vi "FPGA_SICMAutoApproach_v1.vi"() -> ()   [LabVIEW 2021]
uses:
  <vilib>/rvi/eio/common/nirviEmuTemplateMethod_errors.vi
  <vilib>/rvi/Emulation/niFpgaGetClockAttributes.vi
  <vilib>/rvi/Emulation/niFpgaSctlEmulationGetInTimedLoop.vi
  <vilib>/rvi/Emulation/niFpgaEmulationReportErrorSimple.vi
  <vilib>/rvi/Emulation/niFpgaCriticalErrorInLSC.vi
  <vilib>/rvi/Emulation/niFpgaProcessEmulError.vi
  <vilib>/rvi/interface/RandomDataEmulation/niFpgaRandomDataHandleErrors.vi
  <vilib>/rvi/Emulation/niFpgaEmulationIsFPGAContextNoSignature.vi
  <vilib>/rvi/DataTransferAndStorage/Container/Common/niFpgaContainerGetUniqueNameForEmu.vi
  <vilib>/rvi/Memory/Memory_Emulation/niFpgaMemoryEmulationCacheClearOnFirstRun.vi
  <vilib>/rvi/Memory/Memory_Emulation/nirvimemoryEmulationManagerCache_MakeExclusive.vi
  <vilib>/rvi/Memory/Memory_Emulation/niFpgaMemoryEmulationValidateCache.vi
  <vilib>/rvi/Memory/Memory_Emulation/nirvimemoryEmulationManagerCache_InsertValue.vi
  <vilib>/Utility/error.llb/Clear Errors.vi
  <vilib>/rvi/Memory/Memory_Emulation/nirvimemoryEmulationManagerCache_ReleaseExclusive.vi
  <vilib>/rvi/Memory/Memory_Emulation/nirvimemoryEmulationManagerCache_GetValue.vi
  <vilib>/rvi/Memory/Memory_Emulation/nirvimemoryEmulationManagerCache_SetValue.vi
  <vilib>/rvi/occurrence/nirviWaitOnOccurrenceBase.vi
  <vilib>/eio/EIONode/EIONode.xnode
  <vilib>/rvi/FXPMathLib/FxpAdd/XNode/nifxpmath_Add.xnode
  <vilib>/rvi/DataTransferAndStorage/Container/XNode/niFpgaContainer.xnode
  <vilib>/rvi/interface/RandomDataEmulation/nirviRandomDataFpgaReadWriteTemplate.vi
  <vilib>/rvi/DataTransferAndStorage/Register/Emulation/niFpgaRegisterEmulation.vi
  <vilib>/rvi/FXPMathLib/FxpSub/XNode/nifxpmath_Sub.xnode
  <vilib>/rvi/FXPMathLib/sim/FxpSim.dll
panel:
  in  "QuietTime us":u16
  in  "Retract us/step":u32=50
  in  "HoldingElapse us":u32
  in  "SurfaceHold":bool
  out "PeizoFeedbackPos":fxp<+/-,27,5>
  out "PeizoThresholdPos":fxp<+/-,33,17>
  out "PresCurr":fxp<+/-,27,5>
  out "Approached!":bool
  out "ZPeizoPresPos":fxp<+/-,33,17>
  in  "ApproachRate us":u16
  in  "PeizoMax":fxp<+/-,32,16>
  in  "BaselineCurrent":fxp<+/-,32,16>
  in  "stop":bool
  in  "PeizoOffset":fxp<+/-,32,16>
  in  "DeltaMode":bool
  in  "Threshold":fxp<+/-,32,16>
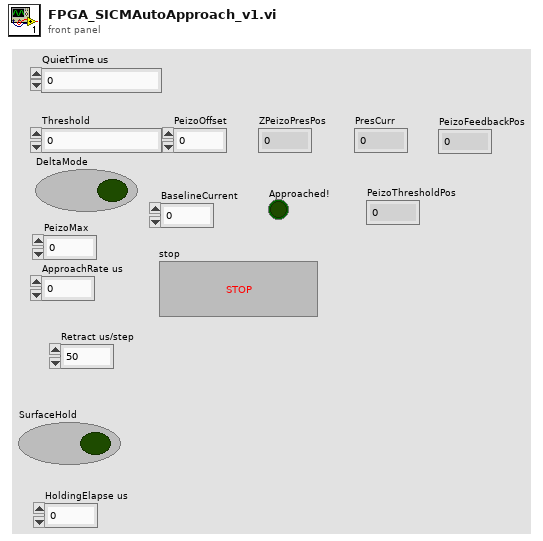
[diagram p1: front panel]
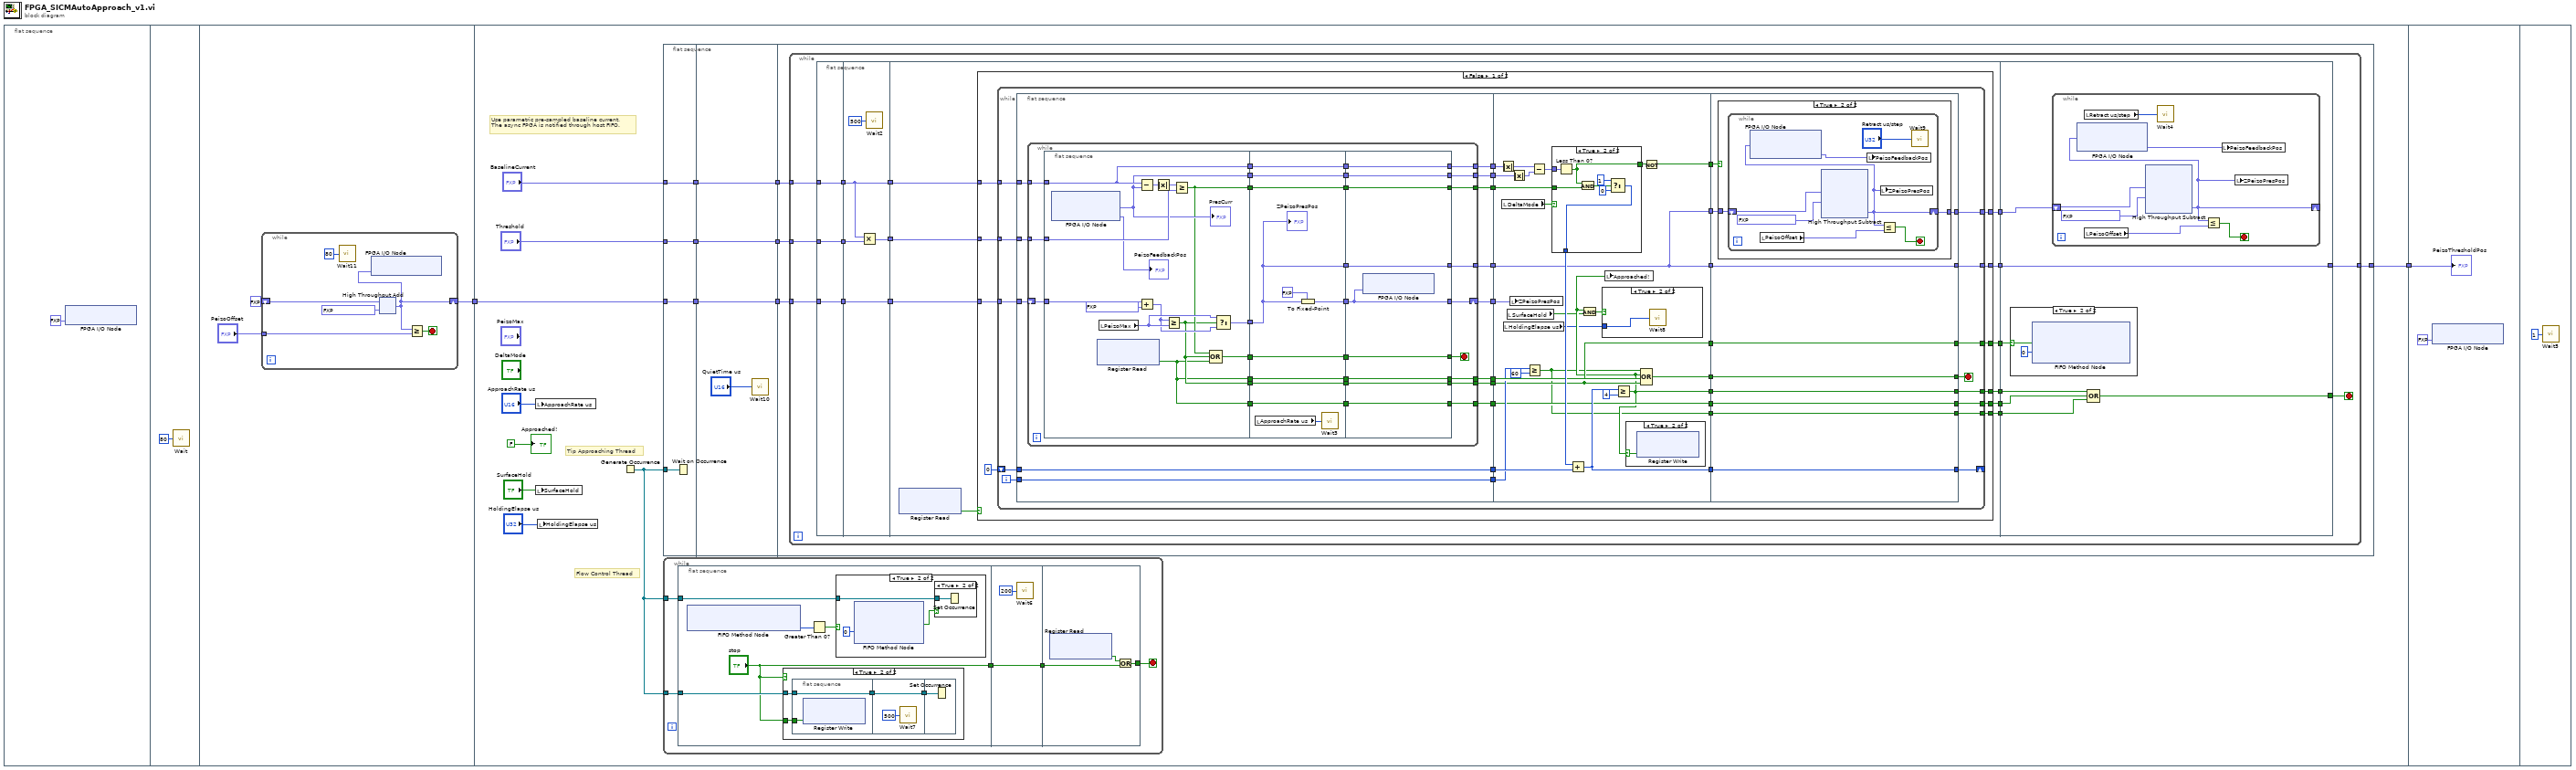
[diagram p0: block diagram]
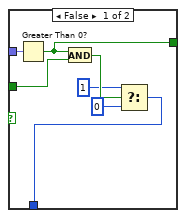
[diagram p4: hidden frame]
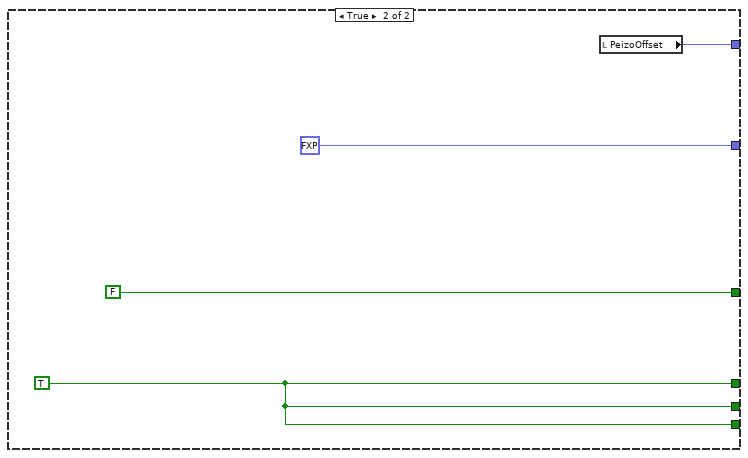
[diagram p6: hidden frame]
diagram:
  n1 = flat-sequence {
    tunnel: [w5] -> w1
    tunnel: [w23] -> w2
    tunnel: w1 -> [w14]
    tunnel: w2 -> [w305]
    frame #0 {
      n2 = xnode "FPGA I/O Node"("Connector0/AO4"=fxp<+/-,20,5> 0.0 ("Connector0/AO2")) -> ()  [unwired: 1 in, 1 out]
    }
    frame #1 {
      n3 = call "Wait"("Count(mSec)"=u8 80) -> ()  [unwired: 1 out]
    }
    frame #2 {
      n4 = while {
        tunnel: "PeizoOffset" -> [w9]
        shift-right: [w10] -> w5
        shift-left: fxp<+/-,48,16> 0.0 -> [w12]
        stop <- w8 stop-if-true
        n5 = call "Wait11"("Count(uSec)"=u32 80) -> ()  [unwired: 1 out]
        n6 = xnode "High Throughput Add"("x"=w12, "y"=fxp<+/-,48,16> 0.00030517578125) -> ("x+y"=w10:fxp<+/-,48,16>)
        n7 = xnode "FPGA I/O Node"("Connector0/AO2"=w10) -> ()  [unwired: 1 in, 1 out]
        n8 = Greater Or Equal?(x=w10, y=w9) -> (x >= y?=w8:bool)
      }
    }
    frame #3 {
      # "Tip Approaching Thread"
      # "Flow Control Thread"
      # "Use parametric pre-sampled baseline current. \nThe async FPGA is notified through host FIFO."
      n9 = local write "ApproachRate us"("ApproachRate us") -> ()
      n10 = local write "SurfaceHold"("SurfaceHold") -> ()
      n11 = local write "HoldingElapse us"("HoldingElapse us") -> ()
      n12 = Generate Occurrence() -> (w28:refnum<k4>)
      n13 = flat-sequence {
        tunnel: "BaselineCurrent" -> [w30]
        tunnel: "Threshold" -> [w31]
        tunnel: w14 -> [w32]
        tunnel: w28 -> [w29]
        tunnel: [w32] -> w17
        tunnel: [w31] -> w16
        tunnel: [w30] -> w15
        tunnel: [w36] -> w20
        tunnel: [w35] -> w19
        tunnel: [w34] -> w18
        tunnel: w17 -> [w36]
        tunnel: w16 -> [w35]
        tunnel: w15 -> [w34]
        tunnel: [w37] -> w23
        tunnel: w20 -> [w40]
        tunnel: w19 -> [w39]
        tunnel: w18 -> [w38]
        frame #0 {
          n14 = Wait on Occurrence(2:w29) -> ()  [unwired: 2 in, 1 out]
        }
        frame #1 {
          n15 = call "Wait10"("Count(uSec)"="QuietTime us") -> ()  [unwired: 1 out]
        }
        frame #2 {
          n16 = while {
            tunnel: w38 -> [w49]
            tunnel: w40 -> [w48]
            tunnel: w39 -> [w47]
            tunnel: [w43] -> w37
            stop <- w51 stop-if-true
            n17 = flat-sequence {
              tunnel: [w60] -> w57
              tunnel: [w59] -> w56
              tunnel: [w58] -> w55
              tunnel: w47 -> [w60]
              tunnel: w48 -> [w58]
              tunnel: w49 -> [w59]
              tunnel: w57 -> [w64]
              tunnel: w56 -> [w63]
              tunnel: [w63] -> w54
              tunnel: w55 -> [w62]
              tunnel: [w62] -> w53
              tunnel: [w61] -> w52
              tunnel: w54 -> [w74]
              tunnel: w53 -> [w73]
              tunnel: w52 -> [w72]
              tunnel: [w71] -> w50
              tunnel: [w70] -> w46
              tunnel: [w69] -> w45
              tunnel: [w68] -> w44
              tunnel: [w67] -> w42
              tunnel: [w66] -> w41
              tunnel: [w266] -> w51
              tunnel: w50 -> [w265]
              tunnel: w46 -> [w267]
              tunnel: w45 -> [w264]
              tunnel: w44 -> [w262]
              tunnel: [w262] -> w43
              tunnel: w42 -> [w263]
              tunnel: w41 -> [w261]
              frame #0 {
              }
              frame #1 {
                n18 = Multiply(x=w63, y=w64) -> (x*y=w61:fxp<+/-,64,32>)
                n19 = call "Wait2"("Count(uSec)"=u16 500) -> ()  [unwired: 1 out]
              }
              frame #2 {
                n20 = xnode ("Register Read")() -> ("Data"=w75:bool)  [unwired: 1 in, 1 out]
                n21 = case shown="False" w75 {
                  tunnel: w74 -> [w85 _]
                  tunnel: w73 -> [w84 _]
                  tunnel: w72 -> [w83 _]
                  tunnel: [w81 w258] -> w71
                  tunnel: [w80 FALSE] -> w70
                  tunnel: [w79 w258] -> w69
                  tunnel: [w78 fxp<+/-,33,17> 0.0 ("PeizoMax")] -> w68
                  tunnel: [w77 w258] -> w67
                  tunnel: [w76 w257] -> w66
                  frame False {
                    n22 = while {
                      tunnel: w85 -> [w116]
                      tunnel: w84 -> [w117]
                      tunnel: w83 -> [w115]
                      shift-right: [w105] -> _
                      shift-left: i16 0 -> [w107]
                      tunnel: [w103] -> w81
                      tunnel: [w96] -> w80
                      tunnel: [w93] -> w79
                      tunnel: [w90] -> w78
                      tunnel: [w88] -> w77
                      tunnel: [w86] -> w76
                      i -> [w109]
                      stop <- w104 stop-if-true
                      n23 = flat-sequence {
                        tunnel: w117 -> [w130]
                        tunnel: w116 -> [w129]
                        tunnel: w115 -> [w128]
                        tunnel: [w127] -> w114
                        tunnel: [w126] -> w113
                        tunnel: [w125] -> w112
                        tunnel: [w124] -> w111
                        tunnel: [w123] -> w110
                        tunnel: w109 -> [w122]
                        tunnel: [w122] -> w108
                        tunnel: w107 -> [w121]
                        tunnel: [w121] -> w106
                        tunnel: [w120] -> w102
                        tunnel: [w119] -> w95
                        tunnel: [w118] -> w92
                        tunnel: w114 -> [w205]
                        tunnel: w113 -> [w211]
                        tunnel: w112 -> [w219]
                        tunnel: w111 -> [w218]
                        tunnel: w110 -> [w215]
                        tunnel: w108 -> [w209]
                        tunnel: w106 -> [w213]
                        tunnel: [w207] -> w101
                        tunnel: [w210] -> w100
                        tunnel: [w200] -> w99
                        tunnel: w102 -> [w202]
                        tunnel: [w203] -> w98
                        tunnel: [w202] -> w97
                        tunnel: w95 -> [w201]
                        tunnel: [w201] -> w94
                        tunnel: w92 -> [w195]
                        tunnel: [w195] -> w91
                        tunnel: [w196] -> w89
                        tunnel: [w195] -> w87
                        tunnel: [w245] -> w104
                        tunnel: [w246] -> w105
                        tunnel: [w244] -> w103
                        tunnel: [w243] -> w96
                        tunnel: w97 -> [w243]
                        tunnel: w98 -> [w242]
                        tunnel: w99 -> [w244]
                        tunnel: w100 -> [w245]
                        tunnel: w101 -> [w246]
                        tunnel: w94 -> [w241]
                        tunnel: [w241] -> w93
                        tunnel: w91 -> [w240]
                        tunnel: [w240] -> w90
                        tunnel: [w239] -> w88
                        tunnel: w89 -> [w239]
                        tunnel: w87 -> [w238]
                        tunnel: [w237] -> w86
                        frame #0 {
                          n24 = while {
                            shift-right: [w155] -> w127
                            shift-left: w130 -> [w159]
                            tunnel: w129 -> [w158]
                            tunnel: w128 -> [w157]
                            tunnel: [w148] -> w126
                            tunnel: [w143] -> w125
                            tunnel: [w142] -> w124
                            tunnel: [w139] -> w123
                            tunnel: [w136] -> w120
                            tunnel: [w133] -> w119
                            tunnel: [w131] -> w118
                            stop <- w151 stop-if-true
                            n25 = flat-sequence {
                              tunnel: w159 -> [w174]
                              tunnel: w158 -> [w165]
                              tunnel: w157 -> [w169]
                              tunnel: [w168] -> w156
                              tunnel: [w167] -> w152
                              tunnel: [w161] -> w149
                              tunnel: [w165] -> w146
                              tunnel: [w164] -> w145
                              tunnel: [w163] -> w140
                              tunnel: [w162] -> w137
                              tunnel: [w161] -> w134
                              tunnel: w156 -> [w175]
                              tunnel: [w184] -> w154
                              tunnel: [w182] -> w153
                              tunnel: w152 -> [w182]
                              tunnel: [w181] -> w150
                              tunnel: w149 -> [w181]
                              tunnel: [w180] -> w147
                              tunnel: w146 -> [w180]
                              tunnel: w145 -> [w179]
                              tunnel: [w179] -> w144
                              tunnel: [w178] -> w141
                              tunnel: w140 -> [w178]
                              tunnel: [w177] -> w138
                              tunnel: w137 -> [w177]
                              tunnel: [w176] -> w135
                              tunnel: w134 -> [w176]
                              tunnel: [w175] -> w132
                              tunnel: [w193] -> w155
                              tunnel: w154 -> [w193]
                              tunnel: w153 -> [w194]
                              tunnel: [w194] -> w151
                              tunnel: [w192] -> w148
                              tunnel: w150 -> [w192]
                              tunnel: [w191] -> w143
                              tunnel: w147 -> [w191]
                              tunnel: [w190] -> w142
                              tunnel: w144 -> [w190]
                              tunnel: [w189] -> w139
                              tunnel: w141 -> [w189]
                              tunnel: [w188] -> w136
                              tunnel: w138 -> [w188]
                              tunnel: [w187] -> w133
                              tunnel: w135 -> [w187]
                              tunnel: [w186] -> w131
                              tunnel: w132 -> [w186]
                              frame #0 {
                                n26 = xnode "FPGA I/O Node"() -> ("Connector0/AI3"=w164:fxp<+/-,27,5>, "Connector0/AI2"=→"PeizoFeedbackPos":fxp<+/-,27,5>)  [unwired: 2 in, 2 out]
                                "PresCurr" <- w164
                                n27 = xnode ("Register Read")() -> ("Data"=w161:bool)  [unwired: 1 in, 1 out]
                                n28 = local read "PeizoMax"() -> (w172:fxp<+/-,32,16>)
                                n29 = Subtract(x=w165, y=w164) -> (x-y=w166:fxp<+/-,39,17>)
                                n30 = Add(x=w174, y=fxp<+/-,32,16> 0.00030517578125) -> (x+y=w171:fxp<+/-,49,17>)
                                n31 = Absolute Value(x=w166) -> (abs(x)=w170:fxp<+,38,16>)
                                n32 = Greater Or Equal?(x=w171, y=w172) -> (x >= y?=w162:bool)
                                n33 = Greater Or Equal?(x=w170, y=w169) -> (x >= y?=w163:bool)
                                n34 = Compound Arithmetic op=OR(w163, w162, w161) -> (w167:bool)
                                n35 = Select(t=w172, s=w162, f=w171) -> (s? t:f=w168:fxp<+/-,49,17>)
                              }
                              frame #1 {
                                n36 = local read "ApproachRate us"() -> (w183:u16)
                                n37 = To Fixed-Point(fixed-point type=fxp<+/-,32,16> 0.0, number=w175) -> (fixed-point=w184:fxp<+/-,32,16>)
                                n38 = call "Wait3"("Count(uSec)"=w183) -> ()  [unwired: 1 out]
                                "ZPeizoPresPos" <- w175
                              }
                              frame #2 {
                                n39 = xnode "FPGA I/O Node"("Connector0/AO2"=w193) -> ()  [unwired: 1 in, 1 out]
                              }
                            }
                          }
                        }
                        frame #1 {
                          n40 = Absolute Value(x=w219) -> (abs(x)=w217:fxp<+,32,16>)
                          n41 = local read "DeltaMode"() -> (w220:bool)
                          n42 = local read "HoldingElapse us"() -> (w197:u32)
                          n43 = local read "SurfaceHold"() -> (w198:bool)
                          n44 = local write "ZPeizoPresPos"(w205) -> ()
                          n45 = Absolute Value(x=w218) -> (abs(x)=w216:fxp<+,27,5>)
                          n46 = Greater Or Equal?(x=w209, y=60) -> (x >= y?=w196:bool)
                          n47 = Subtract(x=w217, y=w216) -> (x-y=w214:fxp<+/-,39,17>)
                          n48 = case shown="True" w220 {
                            tunnel: w215 -> [w228 w235]
                            tunnel: w214 -> [w229 w236]
                            tunnel: [w224 w231] -> w212
                            tunnel: [w223 w230] -> w204
                            frame False {
                              n49 = Greater Than 0?(x=w229) -> (x > 0?=w223:bool)
                              n50 = And(x=w223, y=w228) -> (x .and. y?=w227:bool)
                              n51 = Select(t=i16 1, s=w227, f=i16 0) -> (s? t:f=w224:i16)
                            }
                            frame True {
                              n52 = Less Than 0?(x=w236) -> (x < 0?=w230:bool)
                              n53 = And(x=w230, y=w235) -> (x .and. y?=w234:bool)
                              n54 = Select(t=i16 1, s=w234, f=i16 0) -> (s? t:f=w231:i16)
                            }
                          }
                          n55 = Add(x=w212, y=w213) -> (x+y=w207:i16)
                          n56 = Greater Or Equal?(x=w207, y=i16 4) -> (x >= y?=w200:bool)
                          n57 = And(x=w200, y=w198) -> (x .and. y?=w199:bool)
                          n58 = case shown="True" w199 {
                            tunnel: w197 -> [_ w221]
                            frame False {
                            }
                            frame True {
                              n59 = call "Wait8"("Count(uSec)"=w221) -> ()  [unwired: 1 out]
                            }
                          }
                          n60 = local write "Approached!"(w200) -> ()
                          n61 = case shown="True" w200 {
                            selector: w200 -> [_ w222]
                            frame False {
                            }
                            frame True {
                              n62 = xnode ("Register Write")("Data"=w222) -> ()  [unwired: 1 in, 1 out]
                            }
                          }
                          n63 = Compound Arithmetic op=OR(w196, w200, w211, w202) -> (w210:bool)
                          n64 = Not(x=w204) -> (.not. x?=w203:bool)
                        }
                        frame #2 {
                          n65 = case shown="True" w242 {
                            tunnel: w238 -> [w247 w249]
                            tunnel: [w247 w248] -> w237
                            frame False {
                            }
                            frame True {
                              n66 = while {
                                shift-right: [w251] -> w248
                                shift-left: w249 -> [w253]
                                stop <- w255 stop-if-true
                                n67 = local read "PeizoOffset"() -> (w256:fxp<+/-,32,16>)
                                n68 = xnode "High Throughput Subtract"("x"=w253, "y"=fxp<+/-,32,8> 0.0007171630859375) -> ("x-y"=w251:fxp<+/-,32,8>)
                                n69 = xnode "FPGA I/O Node"("Connector0/AO2"=w251) -> ("Connector0/AI2"=w250:fxp<+/-,27,5>)  [unwired: 2 in, 2 out]
                                n70 = local write "PeizoFeedbackPos"(w250) -> ()
                                n71 = local write "ZPeizoPresPos"(w251) -> ()
                                n72 = Less Or Equal?(x=w251, y=w256) -> (x <= y?=w255:bool)
                                n73 = call "Wait9"("Count(uSec)"="Retract us/step") -> ()  [unwired: 1 out]
                              }
                            }
                          }
                        }
                      }
                    }
                  }
                  frame True {
                    w258 = TRUE
                    n74 = local read "PeizoOffset"() -> (w257:fxp<+/-,32,16>)
                  }
                }
              }
              frame #3 {
                n75 = case shown="True" w267 {
                  selector: w267 -> [_ w276]
                  frame False {
                  }
                  frame True {
                    n76 = xnode ("FIFO Method Node")("Element"=w276, "Timeout"=0) -> ()  [unwired: 1 in, 2 out]
                  }
                }
                n77 = while {
                  shift-right: [w268] -> _
                  shift-left: w261 -> [w271]
                  stop <- w273 stop-if-true
                  n78 = local read "Retract us/step"() -> (w270:u32)
                  n79 = local read "PeizoOffset"() -> (w274:fxp<+/-,32,16>)
                  n80 = xnode "High Throughput Subtract"("x"=w271, "y"=fxp<+/-,32,8> 0.0007171630859375) -> ("x-y"=w268:fxp<+/-,32,8>)
                  n81 = xnode "FPGA I/O Node"("Connector0/AO2"=w268) -> ("Connector0/AI2"=w269:fxp<+/-,27,5>)  [unwired: 2 in, 2 out]
                  n82 = call "Wait4"("Count(uSec)"=w270) -> ()  [unwired: 1 out]
                  n83 = Less Or Equal?(x=w268, y=w274) -> (x <= y?=w273:bool)
                  n84 = local write "PeizoFeedbackPos"(w269) -> ()
                  n85 = local write "ZPeizoPresPos"(w268) -> ()
                }
                n86 = Compound Arithmetic op=OR(w265, w264, w263) -> (w266:bool)
              }
            }
          }
        }
      }
      n87 = while {
        tunnel: w28 -> [w281]
        tunnel: w28 -> [w277]
        stop <- w278 stop-if-true
        n88 = flat-sequence {
          tunnel: w281 -> [w286]
          tunnel: ["stop"] -> w279
          tunnel: w277 -> [w283]
          tunnel: [w300] -> w280
          tunnel: w279 -> [w300]
          tunnel: w280 -> [w304]
          tunnel: [w302] -> w278
          frame #0 {
            n89 = xnode ("FIFO Method Node")() -> ("Number of Elements to Read"=w284:u32)  [unwired: 1 in, 1 out]
            n90 = case shown="True" "stop" {
              tunnel: w283 -> [_ w290]
              tunnel: "stop" -> [_ w289]
              frame False {
              }
              frame True {
                n91 = flat-sequence {
                  tunnel: w290 -> [w292]
                  tunnel: [w292] -> w288
                  tunnel: w289 -> [w291]
                  tunnel: w288 -> [w294]
                  tunnel: [w294] -> w287
                  tunnel: w287 -> [w295]
                  frame #0 {
                    n92 = xnode ("Register Write")("Data"=w291) -> ()  [unwired: 1 in, 1 out]
                  }
                  frame #1 {
                    n93 = call "Wait7"("Count(uSec)"=u16 500) -> ()  [unwired: 1 out]
                  }
                  frame #2 {
                    n94 = Set Occurrence(w295) -> ()
                  }
                }
              }
            }
            n95 = Greater Than 0?(x=w284) -> (x > 0?=w285:bool)
            n96 = case shown="True" w285 {
              tunnel: w286 -> [_ w298]
              frame False {
              }
              frame True {
                n97 = xnode ("FIFO Method Node")("Timeout"=0) -> ("Element"=w296:bool)  [unwired: 1 in, 2 out]
                n98 = case shown="True" w296 {
                  tunnel: w298 -> [_ w299]
                  frame False {
                  }
                  frame True {
                    n99 = Set Occurrence(w299) -> ()
                  }
                }
              }
            }
          }
          frame #1 {
            n100 = call "Wait6"("Count(uSec)"=u16 200) -> ()  [unwired: 1 out]
          }
          frame #2 {
            n101 = xnode ("Register Read")() -> ("Data"=w303:bool)  [unwired: 1 in, 1 out]
            n102 = Or(x=w303, y=w304) -> (x .or. y?=w302:bool)
          }
        }
      }
      "Approached!" <- FALSE
    }
    frame #4 {
      n103 = xnode "FPGA I/O Node"("Connector0/AO2"=fxp<+/-,20,5> 0.0) -> ()  [unwired: 1 in, 1 out]
      "PeizoThresholdPos" <- w305
    }
    frame #5 {
      n104 = call "Wait5"("Count(mSec)"=u8 1) -> ()  [unwired: 1 out]
    }
  }
